vi "V7310.File.Read.vi"(8 "error in":errorcluster, 11 "SettingsPath":path) -> (0 "error out":errorcluster)   [LabVIEW 2016]
uses:
  tools/Tma.lib/nlconfig.llb/fp2ini mode.ctl
  Global/ApplicationGlobal.vi
  V7310.Global.vi
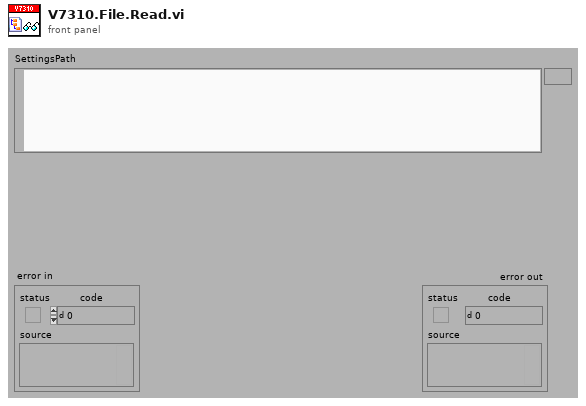
[diagram p1: front panel]
types:
  T1 = typedef "fp2ini mode.ctl" = enum16{"Read Controls", "Write Controls", "Write Indicators", "Read Indicators", "Write all", "Read all"}
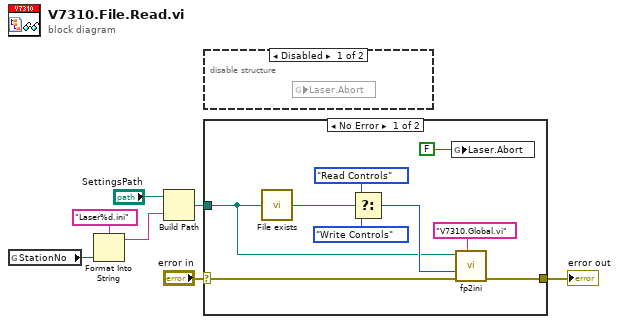
[diagram p0: block diagram]
diagram:
  n1 = global read "ApplicationGlobal.vi" "StationNo"() -> (w3:i32)
  n2 = Format Into String(format string="Laser%d.ini" ("name or relative path"), w3) -> (resulting string=w1:string)  [unwired: 2 in, 1 out]
  n3 = Build Path(base path="SettingsPath", name or relative path=w1) -> (appended path=w7:path)
  n4 = case shown="No Error" "error in" {
    selector: "error in" -> [w16 w17]
    tunnel: [w11 w17] -> w5
    tunnel: w7 -> [w9 _]
    frame No Error {
      n5 = call "File exists.vi"("file path"=w9) -> ("exists?"=w10:bool)  [unwired: 4 in]
      n6 = Select(t=fp2ini_mode."Read Controls" ("mode"), s=w10, f=fp2ini_mode."Write Controls" ("mode")) -> (s? t:f=w13:T1)
      n7 = global write "V7310.Global.vi" "Laser.Abort"(FALSE ("V7310.Abort")) -> ()
      n8 = call "fp2ini.vi"("vi-name (caller if empty)"="V7310.Global.vi", "error in"=w16, "mode"=w13, "ini-file path"=w9) -> ("error out"=w11:errorcluster)  [unwired: 3 in, 4 out]
    }
    frame Error {
    }
  }
  "error out" <- w5
  n9 = disable-structure shown="Disabled" {
    frame Disabled {
      n10 = global read "V7310.Global.vi" "Laser.Abort"() -> ()  [unwired: 1 in]
    }
    frame Enabled {
    }
  }
